vi "Select Project if Launched From Menu.vi"(8 "error in":errorcluster, 11 "Configuration":T1) -> (0 "error out":errorcluster)   [LabVIEW 2013, in "LVTM.lvlib"]
uses:
  LVTM.lvlib
  Controls_LVTM/LVTM_Config_Info.ctl
  Controls_LVTM/View.ctl
  Controls_LVTM/SharedDataDVR.ctl
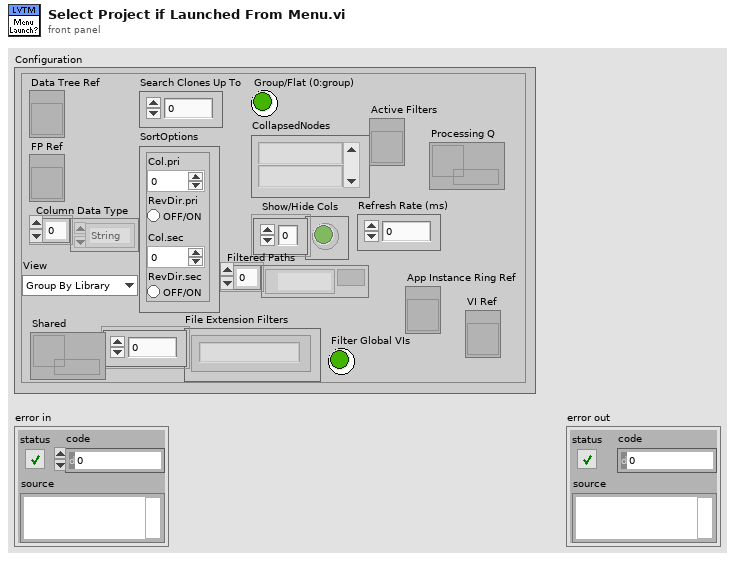
[diagram p1: front panel]
types:
  T1 = typedef "LVTM.lvlib/LVTM_Config_Info.ctl" = cluster{"Data Tree Ref":refnum<vi>, "FP Ref":refnum<vi>, "Column Data Type":enum16{"String", "Numeric"}[], "Search Clones Up To":i32, "SortOptions":cluster{"Col.pri":i32, "RevDir.pri":bool, "Col.sec":i32, "RevDir.sec":bool}, "Group/Flat (0:group)":bool, "CollapsedNodes":string[], "Show/Hide Cols":bool[], "Filtered Paths":path[], "View":T2, "File Extension Filters":string[], "Filter Global VIs":bool, "Shared":refnum<data-value>, "Active Filters":refnum<vi>, "Refresh Rate (ms)":i32, "App Instance Ring Ref":refnum<vi>, "Processing Q":refnum<queue>, "VI Ref":refnum<vi>}
  T2 = typedef "LVTM.lvlib/View.ctl" = enum16{"Group By Library", "Group By Folder", "Flat List"}
  T3 = typedef "LVTM.lvlib/SharedDataDVR.ctl" = cluster{"App":refnum<vi>, "VIs":string[]}
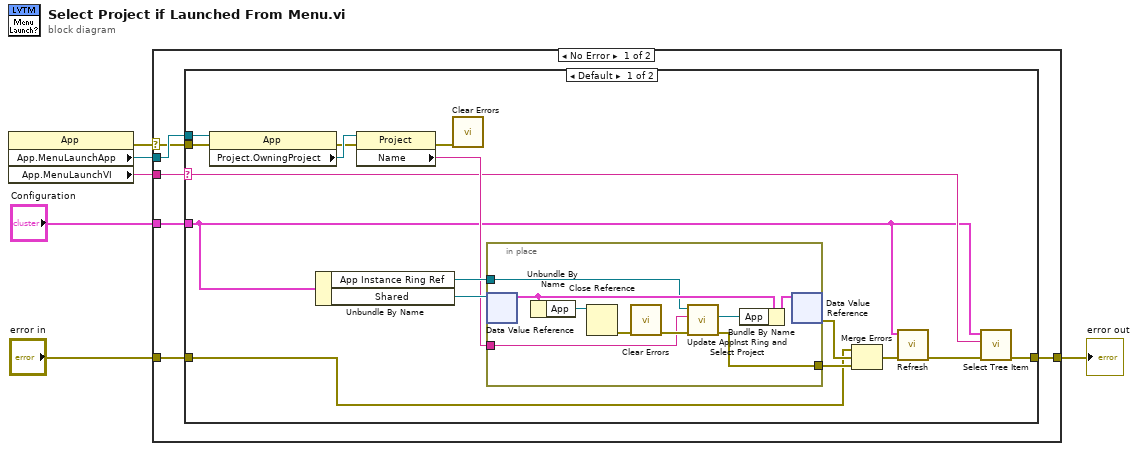
[diagram p0: block diagram]
diagram:
  n1 = property class="App"() -> (error out=w4:errorcluster, "App.MenuLaunchApp"=w6:refnum<vi>, "App.MenuLaunchVI"=w5:string)  [unwired: 2 in, 1 out]
  n2 = case shown="No Error" w4 {
    selector: w4 -> [w10 _]
    tunnel: w6 -> [w12 _]
    tunnel: w5 -> [w11 _]
    tunnel: "Configuration" -> [w9 _]
    tunnel: "error in" -> [w8 w39]
    tunnel: [w7 w39] -> w1
    frame No Error {
      n3 = case shown="Default" w11 {
        selector: w11 -> [w14 _]
        tunnel: w12 -> [w28 _]
        tunnel: w10 -> [w25 _]
        tunnel: w9 -> [w13 _]
        tunnel: w8 -> [w18 w38]
        tunnel: [w15 w38] -> w7
        frame Default {
          n4 = property class="App"(reference=w28, error in=w25) -> (error out=w24:errorcluster, "Project.OwningProject"=w27:refnum<vi>)  [unwired: 1 out]
          n5 = Unbundle By Name(w13) -> ("App Instance Ring Ref"=w19:refnum<vi>, "Shared"=w22:refnum<data-value>)
          n6 = property class="Project"(reference=w27, error in=w24) -> (error out=w26:errorcluster, "Name"=w17:string)  [unwired: 1 out]
          n7 = call <vilib>:"Clear Errors.vi"("error in (no error)"=w26) -> ()  [unwired: 6 in, 1 out]
          n8 = in-place {
            in-place-border: w19 -> [w36]
            in-place-border: [w33] -> w20
            in-place-border: w17 -> [w29]
            n9 = in-place-dvr #1(w22) -> (w37:T3)  [unwired: 1 out]
            n10 = Unbundle By Name(w37) -> ("App"=w32:refnum<vi>)
            n11 = Close Reference(reference=w32) -> (error out=w31:errorcluster)  [unwired: 1 in]
            n12 = call <vilib>:"Clear Errors.vi"("error in (no error)"=w31) -> ("error out"=w30:errorcluster)  [unwired: 6 in]
            n13 = call "Update AppInst Ring and Select Project.vi"("error in"=w30, "Project Name"=w29, "Ring in"=w36) -> ("error out"=w33:errorcluster, "AppInst out"=w34:refnum<vi>)  [unwired: 7 in]
            n14 = Bundle By Name(cluster=w37, "App"=w34) -> (w35:T3)
            n15 = in-place-dvr #1(w35) -> (w21:errorcluster)  [unwired: 1 out]
          }
          n16 = Merge Errors(w18, w21, w20) -> (w23:errorcluster)
          n17 = call "Refresh.vi"("error in (no error)"=w23, "Configuration"=w13) -> ("error out"=w16:errorcluster)  [unwired: 9 in]
          n18 = call "Select Tree Item.vi"("error in"=w16, "Item Tag"=w14, "Configuration"=w13) -> ("error out"=w15:errorcluster)  [unwired: 8 in]
        }
        frame "_ProjectWindow2" {
          # "#ToDo Find way to get the project name from ManuLaunchApp, when launched from the project window."
          # "This was launched from the menu on the project window.\nNot sure how to find the project name from here."
        }
      }
    }
    frame Error {
      # "This was not a menu launch"
    }
  }
  "error out" <- w1
